vi "DimConfig.vi"(8 "error in (no error)":errorcluster, 11 "Dim in":sgl[](array[numeric])) -> (0 "error out":errorcluster, 3 "Dim":sgl[](array[numeric]))   [LabVIEW 2014, in "ConfigProg.lvlib"]
doc: "Configura las dimensiones."
uses:
  ConfigProg.lvlib
panel:
  in  "Stop Dim":bool
  in  "Delete Dim":bool
  in  "Add Dim":bool
  in  "Dimensiones":i32(listbox)=-1
  in  "Cancel Dim":bool
  in  "Save Dim":bool
  in  "Valor:":sgl format="%.6f"
  in  "Edit Dim":bool
  out "Nro Pieza:":string="D1"
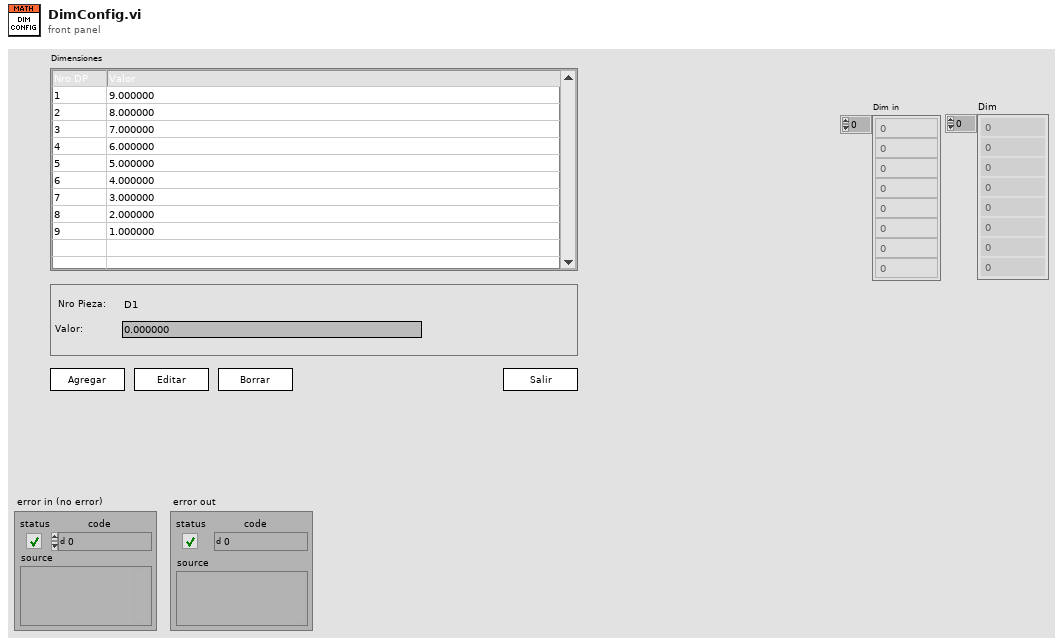
[diagram p1: front panel]
types:
  T1 = enum8{"Enabled", "Disabled", "Disabled and Grayed Out"}
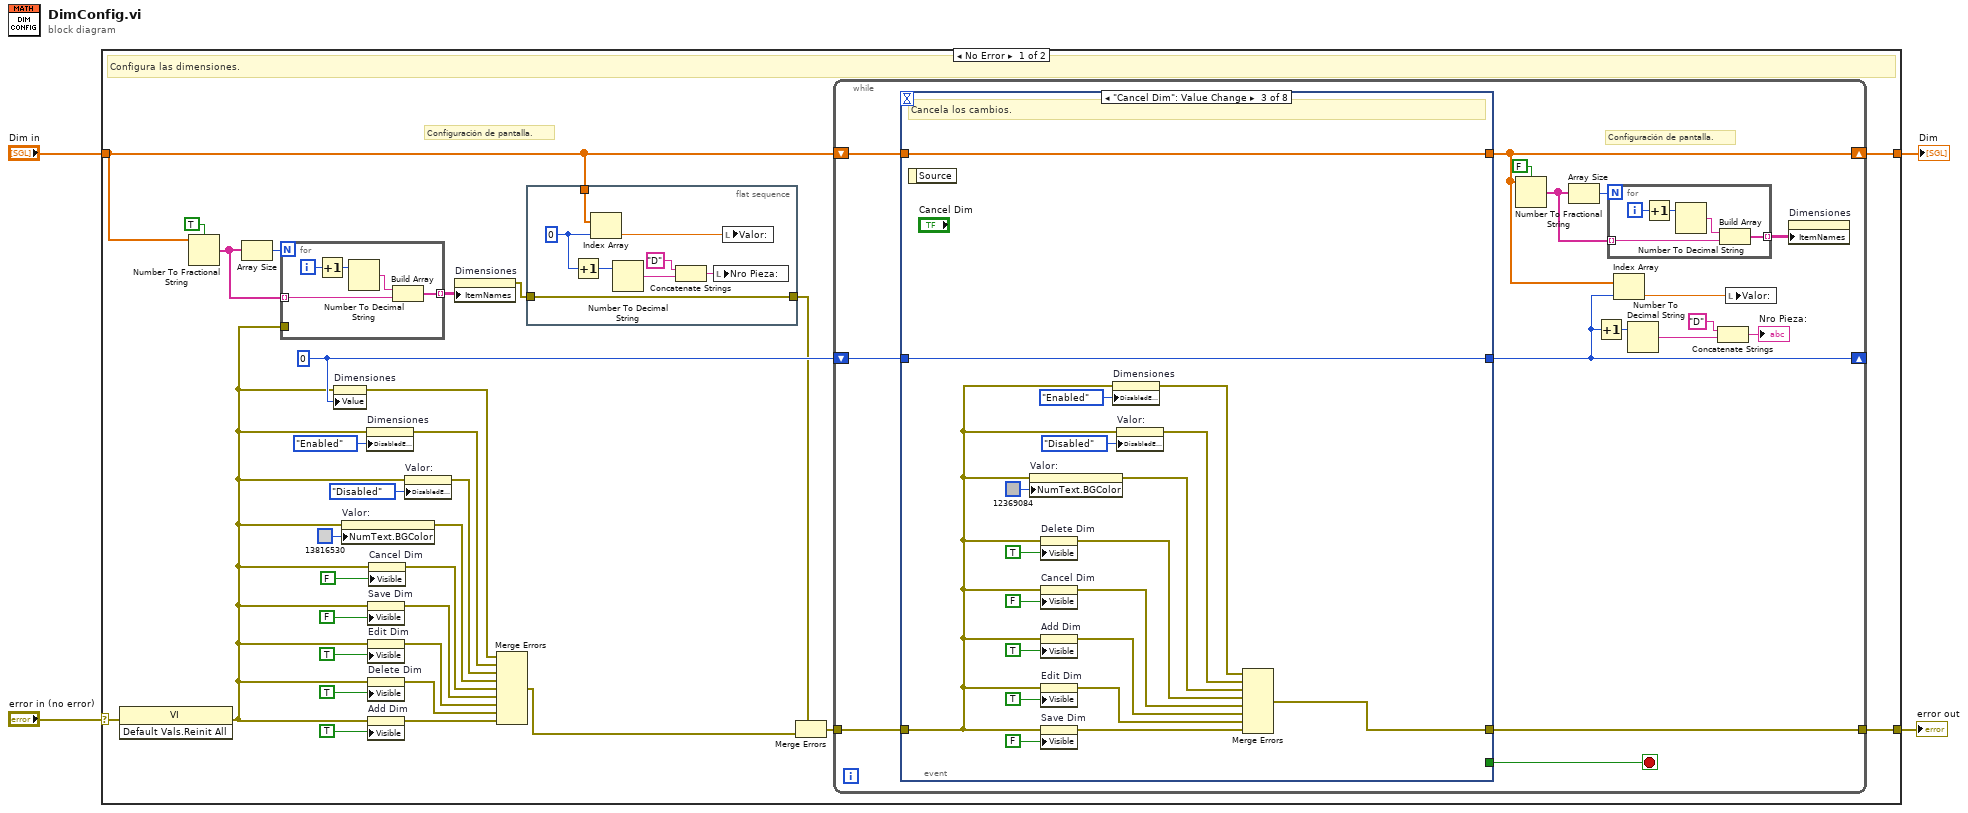
[diagram p0: block diagram]
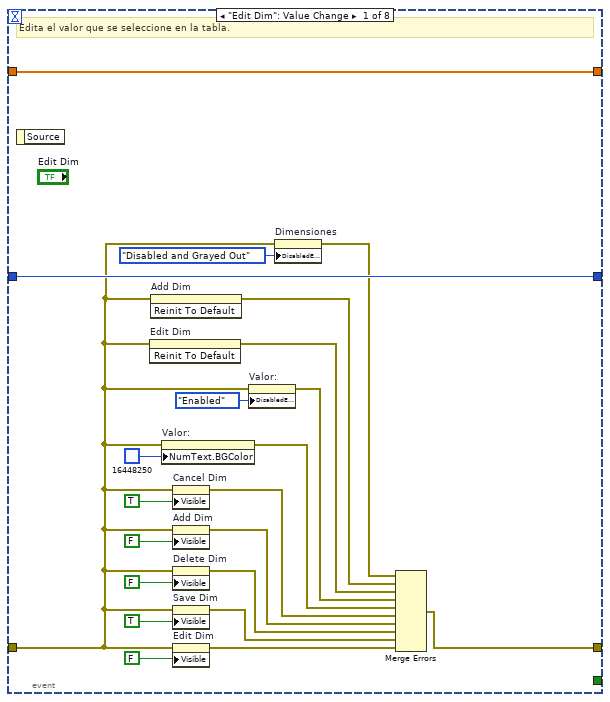
[diagram p2: hidden frame]
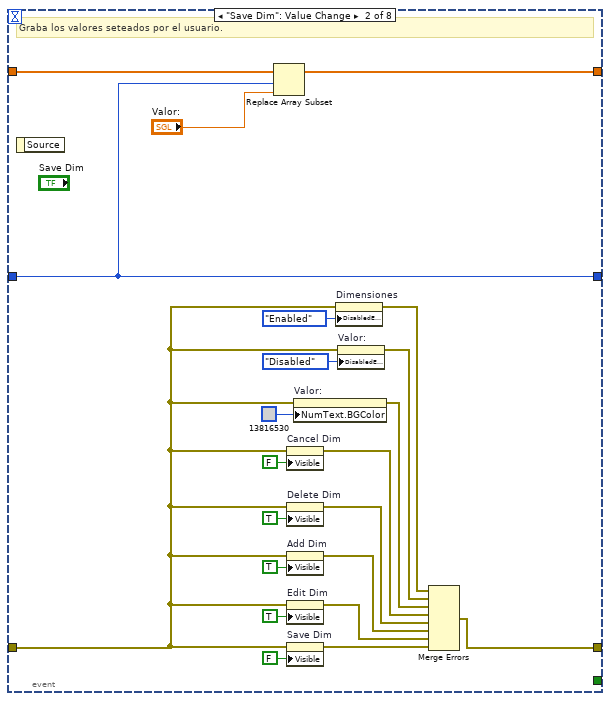
[diagram p3: hidden frame]
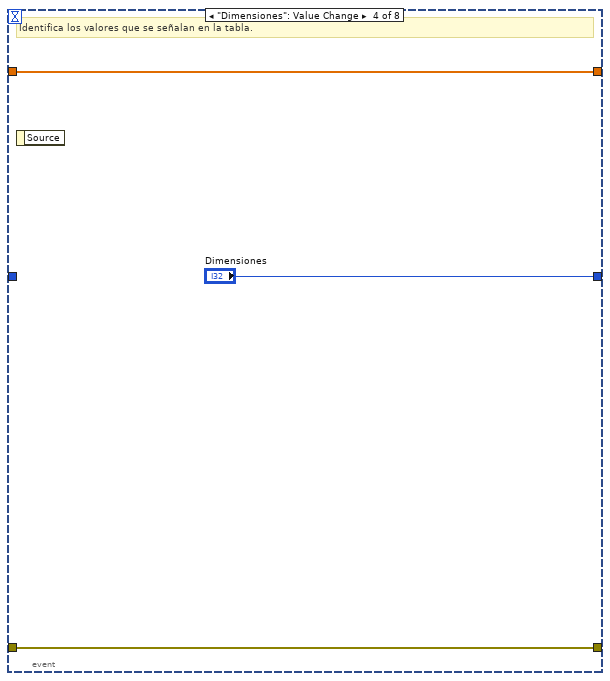
[diagram p4: hidden frame]
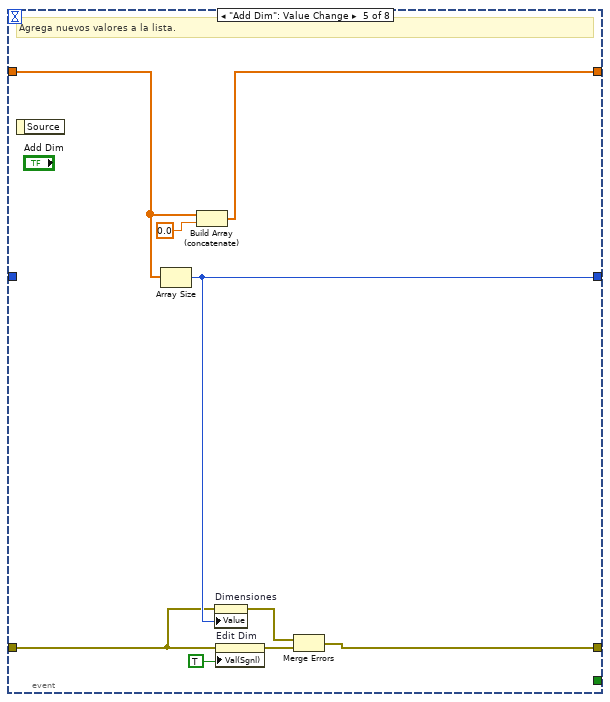
[diagram p5: hidden frame]
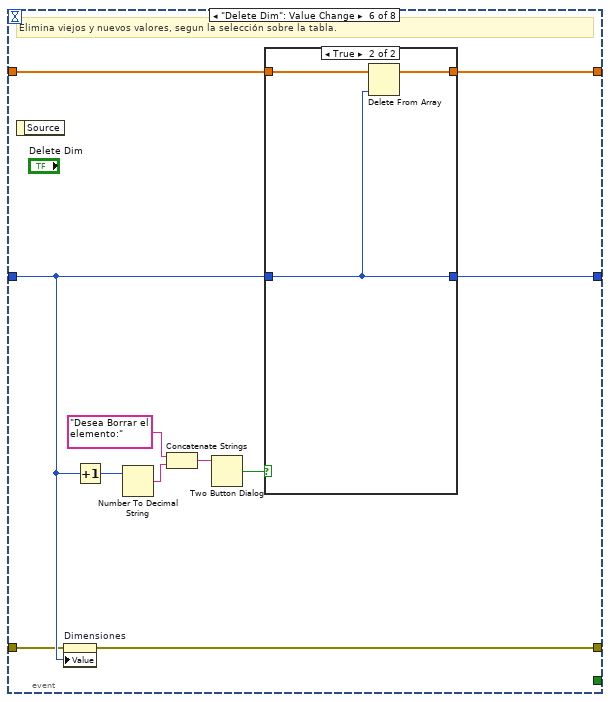
[diagram p6: hidden frame]
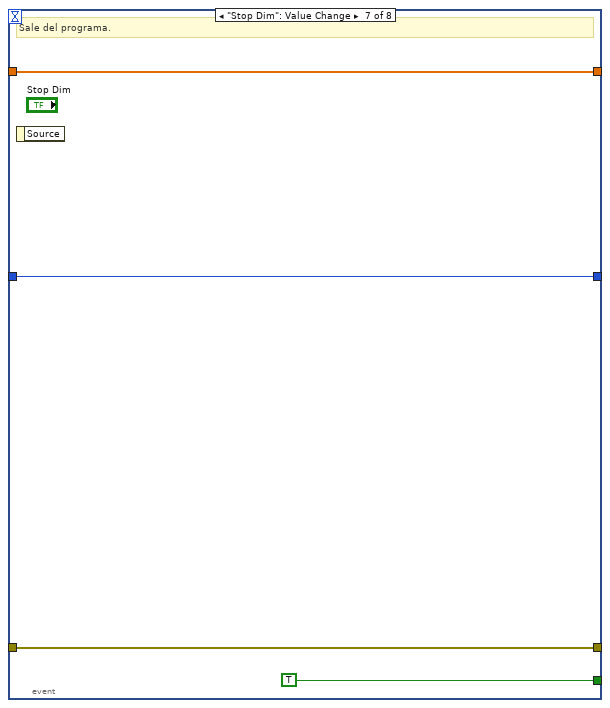
[diagram p8: hidden frame]
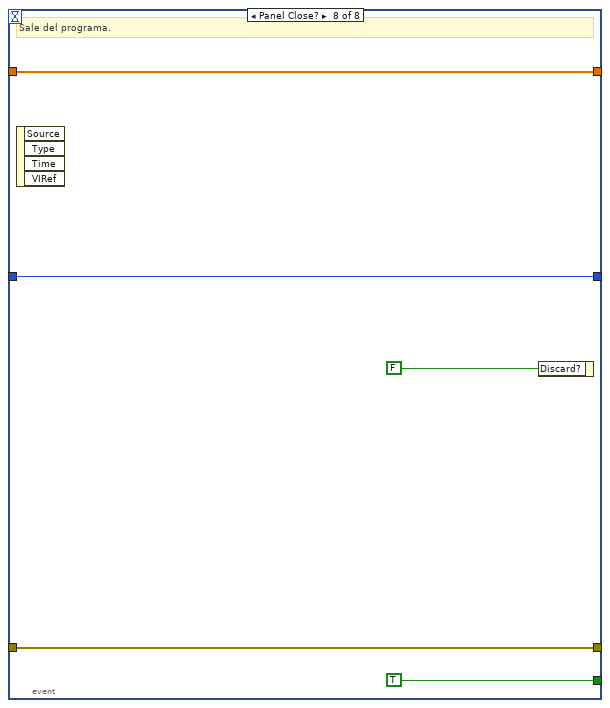
[diagram p9: hidden frame]
diagram:
  n1 = case shown="No Error" "error in (no error)" {
    selector: "error in (no error)" -> [w5 w171]
    tunnel: [w35 w171] -> w4
    tunnel: [w19 w172] -> w3
    tunnel: "Dim in" -> [w6 w172]
    frame No Error {
      w27 = 0 ("disabled index (col)")
      # "Configuración de pantalla."
      # "Configura las dimensiones."
      n2 = invoke class="VI" method="Default Vals.Reinit All"(error in=w5) -> (error out=w8:errorcluster)  [unwired: 2 in, 2 out]
      n3 = Number To Fractional String(use system decimal point (T)=TRUE, number=w6) -> (F-format string=w18:string[])  [unwired: 2 in]
      n4 = Array Size(array=w18) -> (size(s)=w29:i32)
      n5 = for {
        N: w29 -> [_]
        tunnel: w18 -> [w48] mode=indexing
        tunnel: [w46] -> w28 mode=indexing
        tunnel: w8 -> [_]
        i -> [w44]
        n6 = Increment(x=w44) -> (x+1=w45:i32)
        n7 = Number To Decimal String(number=w45) -> (decimal integer string=w47:string)  [unwired: 1 in]
        n8 = Build Array(w47, w48) -> (w46:string[])
      }
      n9 = property on="Dimensiones" class="MCListbox (strict)"(error in=w8, "Value"=w27) -> (error out=w7:errorcluster)  [unwired: 1 in, 1 out]
      n10 = property on="Valor:" class="DigNum (strict)"(error in=w8, "NumText.BGColor"=u32 13816530) -> (error out=w25:errorcluster)  [unwired: 1 in, 1 out]
      n11 = property on="Dimensiones" class="MCListbox (strict)"(error in=w8, "DisabledEnum"=T1."Enabled" ("Disabled")) -> (error out=w9:errorcluster)  [unwired: 1 in, 1 out]
      n12 = property on="Save Dim" class="Bool"(error in=w8, "Visible"=FALSE) -> (error out=w32:errorcluster)  [unwired: 1 in, 1 out]
      n13 = property on="Edit Dim" class="Bool (strict)"(error in=w8, "Visible"=TRUE) -> (error out=w31:errorcluster)  [unwired: 1 in, 1 out]
      n14 = property on="Delete Dim" class="Bool"(error in=w8, "Visible"=TRUE) -> (error out=w22:errorcluster)  [unwired: 1 in, 1 out]
      n15 = property on="Add Dim" class="Bool (strict)"(error in=w8, "Visible"=TRUE) -> (error out=w20:errorcluster)  [unwired: 1 in, 1 out]
      n16 = property on="Cancel Dim" class="Bool"(error in=w8, "Visible"=FALSE) -> (error out=w24:errorcluster)  [unwired: 1 in, 1 out]
      n17 = property on="Valor:" class="DigNum (strict)"(error in=w8, "DisabledEnum"=T1."Disabled" ("Disabled")) -> (error out=w15:errorcluster)  [unwired: 1 in, 1 out]
      n18 = property on="Dimensiones" class="MCListbox (strict)"("ItemNames"=w28) -> (error out=w14:errorcluster)  [unwired: 2 in, 1 out]
      n19 = Merge Errors(w7, w9, w15, w25, w24, w32, w31, w22, w20) -> (w12:errorcluster)
      n20 = flat-sequence {
        tunnel: w6 -> [w39]
        tunnel: [w36] -> w11
        tunnel: w14 -> [w36]
        frame #0 {
          w38 = 0 ("disabled index (col)")
          n21 = Increment(x=w38) -> (x+1=w42:i32)
          n22 = Index Array(array=w39, index=w38) -> (element=w40:sgl)
          n23 = Number To Decimal String(number=w42) -> (decimal integer string=w43:string)  [unwired: 1 in]
          n24 = Concatenate Strings("D" ("string"), w43) -> (w37:string)
          n25 = local write "Nro Pieza:"(w37) -> ()
          n26 = local write "Valor:"(w40) -> ()
        }
      }
      n27 = Merge Errors(w11, w12) -> (w13:errorcluster)
      n28 = while {
        shift-right: [w52] -> w19
        shift-left: w6 -> [w62]
        shift-right: [w60] -> _
        shift-left: w27 -> [w61]
        tunnel: w13 -> [w49]
        tunnel: [w64] -> w35
        stop <- w63 stop-if-true
        # "Configuración de pantalla."
        n29 = event shown="[2] \"Cancel Dim\": Value Change" {
          selector: _ -> [_ _ _ _ _ _ _ _]
          dyn-events: _ -> [_ _ _ _ _ _ _ _]
          timeout: _ -> [_ _ _ _ _ _ _ _]
          tunnel: w62 -> [w85 w106 w133 w136 w142 w154 w164 w170]
          tunnel: [w85 w105 w133 w136 w145 w153 w164 w170] -> w52
          tunnel: [w84 w107 w132 "Dimensiones" w141 w155 w163 w169] -> w60
          tunnel: w61 -> [w84 w107 w132 _ _ w148 w163 w169]
          tunnel: w49 -> [w70 w92 w114 w134 w138 w147 w165 w167]
          tunnel: [w86 w108 w124 w134 w137 w146 w165 w167] -> w64
          tunnel: [_ _ _ _ _ _ TRUE ("Stop Dim") TRUE ("Stop Dim")] -> w63
          event "Edit Dim": Value Change {
            # "Edita el valor que se seleccione en la tabla."
            n30 = event-data() -> ()  [unwired: 1 in, 1 out]
            n31 = invoke on="Edit Dim" class="Bool (strict)" method="Reinit To Default"(error in=w70) -> (error out=w75:errorcluster)  [unwired: 2 in, 2 out]
            n32 = invoke on="Add Dim" class="Bool (strict)" method="Reinit To Default"(error in=w70) -> (error out=w76:errorcluster)  [unwired: 2 in, 2 out]
            n33 = property on="Valor:" class="DigNum (strict)"(error in=w70, "NumText.BGColor"=u32 16448250) -> (error out=w78:errorcluster)  [unwired: 1 in, 1 out]
            n34 = property on="Cancel Dim" class="Bool"(error in=w70, "Visible"=TRUE) -> (error out=w77:errorcluster)  [unwired: 1 in, 1 out]
            n35 = property on="Add Dim" class="Bool (strict)"(error in=w70, "Visible"=FALSE) -> (error out=w80:errorcluster)  [unwired: 1 in, 1 out]
            n36 = property on="Delete Dim" class="Bool"(error in=w70, "Visible"=FALSE) -> (error out=w82:errorcluster)  [unwired: 1 in, 1 out]
            n37 = property on="Save Dim" class="Bool"(error in=w70, "Visible"=TRUE) -> (error out=w87:errorcluster)  [unwired: 1 in, 1 out]
            n38 = property on="Edit Dim" class="Bool (strict)"(error in=w70, "Visible"=FALSE) -> (error out=w91:errorcluster)  [unwired: 1 in, 1 out]
            n39 = property on="Valor:" class="DigNum (strict)"(error in=w70, "DisabledEnum"=T1."Enabled" ("Disabled")) -> (error out=w73:errorcluster)  [unwired: 1 in, 1 out]
            n40 = property on="Dimensiones" class="MCListbox (strict)"(error in=w70, "DisabledEnum"=T1."Disabled and Grayed Out" ("Disabled")) -> (error out=w71:errorcluster)  [unwired: 1 in, 1 out]
            n41 = Merge Errors(w71, w76, w75, w73, w78, w77, w80, w82, w87, w91) -> (w86:errorcluster)
          }
          event "Save Dim": Value Change {
            # "Graba los valores seteados por el usuario."
            n42 = event-data() -> ()  [unwired: 1 in, 1 out]
            n43 = Replace Array Subset(array=w106, new element="Valor:", index=w107) -> (w105:sgl[])
            n44 = property on="Cancel Dim" class="Bool"(error in=w92, "Visible"=FALSE) -> (error out=w100:errorcluster)  [unwired: 1 in, 1 out]
            n45 = property on="Delete Dim" class="Bool"(error in=w92, "Visible"=TRUE) -> (error out=w99:errorcluster)  [unwired: 1 in, 1 out]
            n46 = property on="Add Dim" class="Bool (strict)"(error in=w92, "Visible"=TRUE) -> (error out=w103:errorcluster)  [unwired: 1 in, 1 out]
            n47 = property on="Edit Dim" class="Bool (strict)"(error in=w92, "Visible"=TRUE) -> (error out=w113:errorcluster)  [unwired: 1 in, 1 out]
            n48 = property on="Save Dim" class="Bool"(error in=w92, "Visible"=FALSE) -> (error out=w112:errorcluster)  [unwired: 1 in, 1 out]
            n49 = property on="Valor:" class="DigNum (strict)"(error in=w92, "NumText.BGColor"=u32 13816530) -> (error out=w98:errorcluster)  [unwired: 1 in, 1 out]
            n50 = property on="Dimensiones" class="MCListbox (strict)"(error in=w92, "DisabledEnum"=T1."Enabled" ("Disabled")) -> (error out=w93:errorcluster)  [unwired: 1 in, 1 out]
            n51 = property on="Valor:" class="DigNum (strict)"(error in=w92, "DisabledEnum"=T1."Disabled" ("Disabled")) -> (error out=w95:errorcluster)  [unwired: 1 in, 1 out]
            n52 = Merge Errors(w93, w95, w98, w100, w99, w103, w113, w112) -> (w108:errorcluster)
          }
          event "Cancel Dim": Value Change {
            # "Cancela los cambios."
            n53 = event-data() -> ()  [unwired: 1 in, 1 out]
            n54 = property on="Valor:" class="DigNum (strict)"(error in=w114, "NumText.BGColor"=u32 12369084) -> (error out=w121:errorcluster)  [unwired: 1 in, 1 out]
            n55 = property on="Delete Dim" class="Bool"(error in=w114, "Visible"=TRUE) -> (error out=w120:errorcluster)  [unwired: 1 in, 1 out]
            n56 = property on="Cancel Dim" class="Bool"(error in=w114, "Visible"=FALSE) -> (error out=w119:errorcluster)  [unwired: 1 in, 1 out]
            n57 = property on="Add Dim" class="Bool (strict)"(error in=w114, "Visible"=TRUE) -> (error out=w125:errorcluster)  [unwired: 1 in, 1 out]
            n58 = property on="Edit Dim" class="Bool (strict)"(error in=w114, "Visible"=TRUE) -> (error out=w131:errorcluster)  [unwired: 1 in, 1 out]
            n59 = property on="Save Dim" class="Bool"(error in=w114, "Visible"=FALSE) -> (error out=w130:errorcluster)  [unwired: 1 in, 1 out]
            n60 = property on="Dimensiones" class="MCListbox (strict)"(error in=w114, "DisabledEnum"=T1."Enabled" ("Disabled")) -> (error out=w115:errorcluster)  [unwired: 1 in, 1 out]
            n61 = property on="Valor:" class="DigNum (strict)"(error in=w114, "DisabledEnum"=T1."Disabled" ("Disabled")) -> (error out=w117:errorcluster)  [unwired: 1 in, 1 out]
            n62 = Merge Errors(w115, w117, w121, w120, w119, w125, w131, w130) -> (w124:errorcluster)
          }
          event "Dimensiones": Value Change {
            # "Identifica los valores que se señalan en la tabla."
            n63 = event-data() -> ()  [unwired: 1 in, 1 out]
          }
          event "Add Dim": Value Change {
            # "Agrega nuevos valores a la lista."
            n64 = event-data() -> ()  [unwired: 1 in, 1 out]
            n65 = Array Size(array=w142) -> (size(s)=w141:i32)
            n66 = Build Array (concatenate)(w142, sgl 0.0) -> (w145:sgl[])
            n67 = property on="Dimensiones" class="MCListbox (strict)"(error in=w138, "Value"=w141) -> (error out=w140:errorcluster)  [unwired: 1 in, 1 out]
            n68 = property on="Edit Dim" class="Bool (strict)"(error in=w138, "Val(Sgnl)"=TRUE) -> (error out=w139:errorcluster)  [unwired: 1 in, 1 out]
            n69 = Merge Errors(w140, w139) -> (w137:errorcluster)
          }
          event "Delete Dim": Value Change {
            # "Elimina viejos y nuevos valores, segun la selección sobre la tabla."
            n70 = event-data() -> ()  [unwired: 1 in, 1 out]
            n71 = property on="Dimensiones" class="MCListbox (strict)"(error in=w147, "Value"=w148) -> (error out=w146:errorcluster)  [unwired: 1 in, 1 out]
            n72 = Increment(x=w148) -> (x+1=w149:i32)
            n73 = Number To Decimal String(number=w149) -> (decimal integer string=w151:string)  [unwired: 1 in]
            n74 = Concatenate Strings("Desea Borrar el elemento:" ("message"), w151) -> (w150:string)
            n75 = Two Button Dialog(message=w150) -> (T button?=w156:bool)  [unwired: 2 in]
            n76 = case shown="True" w156 {
              tunnel: w154 -> [w157 w161]
              tunnel: [w158 w159] -> w155
              tunnel: w148 -> [w158 w159]
              tunnel: [w157 w160] -> w153
              frame False {
              }
              frame True {
                n77 = Delete From Array(array=w161, index=w159) -> (array with subset deleted=w160:sgl[])  [unwired: 1 in, 1 out]
              }
            }
          }
          event "Stop Dim": Value Change {
            # "Sale del programa."
            n78 = event-data() -> ()  [unwired: 1 in, 1 out]
          }
          event Panel Close? {
            # "Sale del programa."
            n79 = event-data() -> ()  [unwired: 1 in, 4 out]
            n80 = event-data("Discard?"=FALSE) -> ()  [unwired: 1 in, 1 out]
          }
        }
        n81 = Number To Fractional String(use system decimal point (T)=FALSE, number=w52) -> (F-format string=w53:string[])  [unwired: 2 in]
        n82 = Array Size(array=w53) -> (size(s)=w59:i32)
        n83 = Increment(x=w60) -> (x+1=w56:i32)
        n84 = for {
          N: w59 -> [_]
          tunnel: w53 -> [w69] mode=indexing
          tunnel: [w67] -> w58 mode=indexing
          i -> [w65]
          n85 = Increment(x=w65) -> (x+1=w66:i32)
          n86 = Number To Decimal String(number=w66) -> (decimal integer string=w68:string)  [unwired: 1 in]
          n87 = Build Array(w68, w69) -> (w67:string[])
        }
        n88 = Index Array(array=w52, index=w60) -> (element=w51:sgl)
        n89 = Number To Decimal String(number=w56) -> (decimal integer string=w57:string)  [unwired: 1 in]
        n90 = Concatenate Strings("D" ("string"), w57) -> (→"Nro Pieza:":string)
        n91 = local write "Valor:"(w51) -> ()
        n92 = property on="Dimensiones" class="MCListbox (strict)"("ItemNames"=w58) -> ()  [unwired: 2 in, 2 out]
      }
    }
    frame Error {
    }
  }
  "error out" <- w4
  "Dim" <- w3
